vi "Output.vi"(8 "error in (no error)":errorcluster, 10 "SendCMD":bool, 11 "ReadOnlyIIn":T1={"Qref"={"ValveCTR"=refnum, "Error"=refnum}, "UI_EN"=FALSE, "UserEventREF"={"TimeBasedProducer"={"Reg"=refnum, "Ref"=refnum}, "TimeBasedTempRead"={"Reg"=refnum, "Ref"=refnum}}, "UI_REF"=variant, "Paths"={"Log_Dir"=path "", "TempLog"=path "", "WateringLog"=path "", "Error"=path "", "Settings_Dir"=path "", "CFG.ini"=path "", "Plant_Digital_OP"=path "", "TimeTable"=path "", "Consol_Dir"=path "", "Input"=path "", "Output"=path "", "Timeout"=path "", "TimeoutTable"=path "", "Ch_Stat"=path "", "Temp"=path ""}, "PI_REF"={"IO"=enum."Remote", "Interface"=enum."Serial", "LINX Device Config"={"Interface"=enum."Serial", "COM Port"="COM13", "TCP Configuration"={"IP Address"="", "Port"=0}, "Device Family"=1, "Device ID"=1, "Device Name"="myRIO-1900", "TCP Ref"=refnum, "Channels"={"DI"=[0, 1, 2, 3, 4, 5, 6, 7, 8, 9, 10, 11, 12, 13, 14, 15, 16, 17, 18, 19, 20, 21, 22, 23, 24, 25, 26, 27, 28, 29, 30, 31, 32, 33, 34, 35, 36, 37, 38, 39, 40, 41, 42, 43, 44, 45, 46], "DO"=[0, 1, 2, 3, 4, 5, 6, 7, 8, 9, 10, 11, 12, 13, 14, 15, 16, 17, 18, 19, 20, 21, 22, 23, 24, 25, 26, 27, 28, 29, 30, 31, 32, 33, 34, 35, 36, 37, 38, 39, 40, 41, 42, 43, 44, 45, 46], "AI"=[0, 1, 2, 3, 4, 5, 6, 7, 8, 9, 10, 11], "AO"=[], "PWM"=[3, 5, 6, 9, 10], "QE"=[], "UART"=[0, 1], "I2C 2"=[0], "SPI"=[0], "CAN"=[], "Servo"=[], "AI Ref (V)"=0.0, "AI Resolution (Bits)"=0, "AO Ref (V)"=0.0, "AO Resolution (Bits)"=0}}}, "CFG"={"ProducerEn_PC"=FALSE, "Producer_PC_ms"=0, "ProducerEn_PI"=FALSE, "Producer_PI_ms"=0, "TempLogInterval"=15, "SystemResetTime"=0.0}} {"CFG"."SystemResetTime" format="%<%H:%M:%S>t"}) -> (0 "error out":errorcluster)   [LabVIEW 2014, in "Main.lvlib"]
uses:
  Main.lvlib
  TypeDef/ReadOnly.ctl
  ValveCTRL/TypeDef/Queue_Cluster.ctl
  ValveCTRL/TypeDef/States_Enum.ctl
  ValveCTRL/TypeDef/CHs_List.ctl
  TypeDef/EventData.ctl
  <vilib>/MakerHub/LINX/Private/Type Defs/LINX Ref.ctl
  <vilib>/MakerHub/LINX/Private/Type Defs/Platform.ctl
  <vilib>/MakerHub/LINX/Private/Type Defs/Interface.ctl
  <vilib>/MakerHub/LINX/Private/Device/Type Defs/LINX Device Config.ctl
  <vilib>/MakerHub/LINX/Private/Device/Type Defs/TCP Config.ctl
  <vilib>/MakerHub/LINX/Private/Device/Type Defs/Channels.ctl
  Init/ReadInitCFG/TypeDef/CFG_Cluster.ctl
  ValveCTRL/ValveCTRL.lvlib
  <vilib>/MakerHub/LINX/LMH-LINX.lvlib
  <vilib>/MakerHub/LINX/Private/Device/Device.lvlib
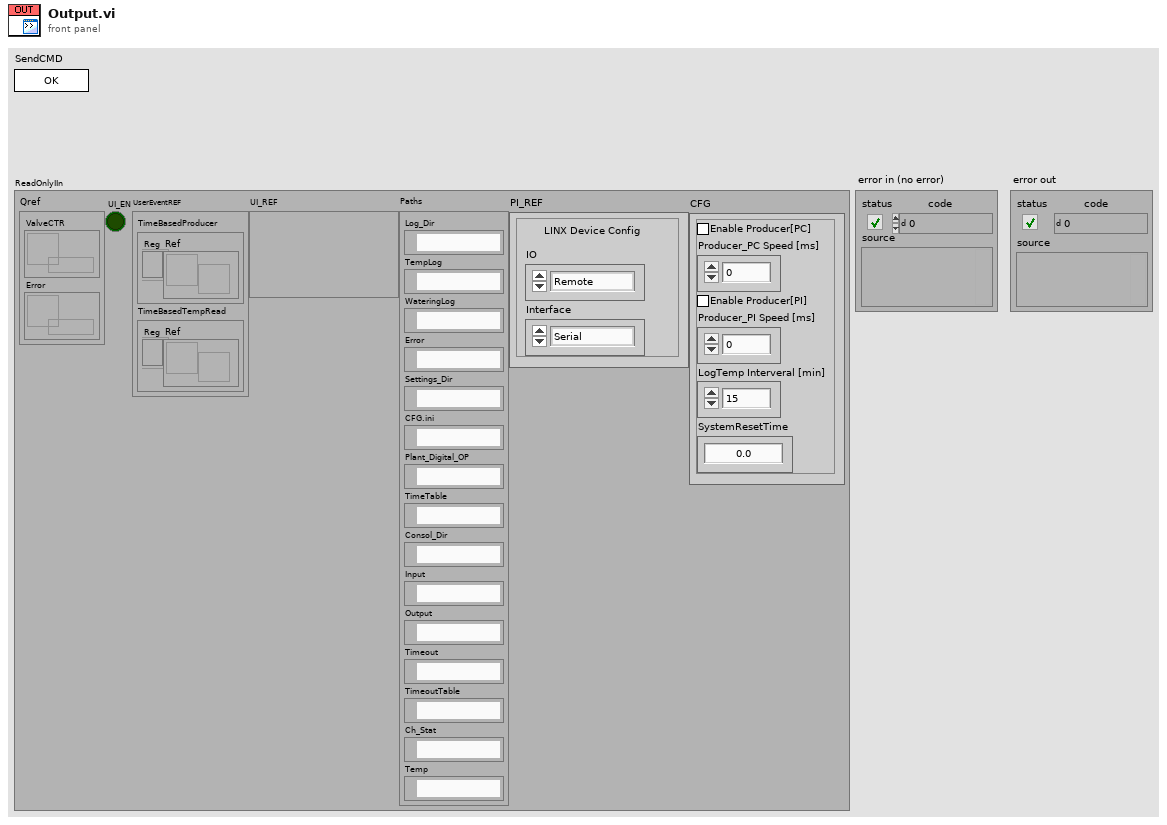
[diagram p1: front panel]
types:
  T1 = typedef "Main.lvlib/ReadOnly.ctl" = cluster{"Qref":cluster{"ValveCTR":refnum<queue>, "Error":refnum<queue>}, "UI_EN":bool, "UserEventREF":cluster{"TimeBasedProducer":cluster{"Reg":refnum<event-registration>, "Ref":refnum<user-event>}, "TimeBasedTempRead":cluster{"Reg":refnum<event-registration>, "Ref":refnum<user-event>}}, "UI_REF":variant, "Paths":cluster{"Log_Dir":path, "TempLog":path, "WateringLog":path, "Error":path, "Settings_Dir":path, "CFG.ini":path, "Plant_Digital_OP":path, "TimeTable":path, "Consol_Dir":path, "Input":path, "Output":path, "Timeout":path, "TimeoutTable":path, "Ch_Stat":path, "Temp":path}, "PI_REF":T2, "CFG":T8}
  T2 = typedef "LMH-LINX.lvlib/LINX Ref.ctl" = cluster{"IO":T3, "Interface":T4, "LINX Device Config":T5}
  T3 = typedef "LMH-LINX.lvlib/Platform.ctl" = enum16{"Remote", "Local"}
  T4 = typedef "LMH-LINX.lvlib/Interface.ctl" = enum16{"Serial", "TCP"}
  T5 = typedef "LMH-LINX.lvlib/Device.lvlib/LINX Device Config.ctl" = cluster{"Interface":T4, "COM Port":refnum<visa-resource-name>, "TCP Configuration":T6, "Device Family":u8, "Device ID":u8, "Device Name":string, "TCP Ref":refnum<k5>, "Channels":T7}
  T6 = typedef "LMH-LINX.lvlib/Device.lvlib/TCP Config.ctl" = cluster{"IP Address":string, "Port":u16}
  T7 = typedef "LMH-LINX.lvlib/Channels.ctl" = cluster{"DI":u8[], "DO":u8[], "AI":u8[], "AO":u8[], "PWM":u8[], "QE":u8[], "UART":u8[], "I2C 2":u8[], "SPI":u8[], "CAN":u8[], "Servo":u8[], "AI Ref (V)":dbl, "AI Resolution (Bits)":u8, "AO Ref (V)":dbl, "AO Resolution (Bits)":u8}
  T8 = typedef "Main.lvlib/CFG_Cluster.ctl" = cluster{"ProducerEn_PC":bool, "Producer_PC_ms":u32, "ProducerEn_PI":bool, "Producer_PI_ms":u32, "TempLogInterval":u32, "SystemResetTime":dbl}
  T9 = enum16{"open", "replace", "create", "open or create", "replace or create", "replace or create with confirmation"}
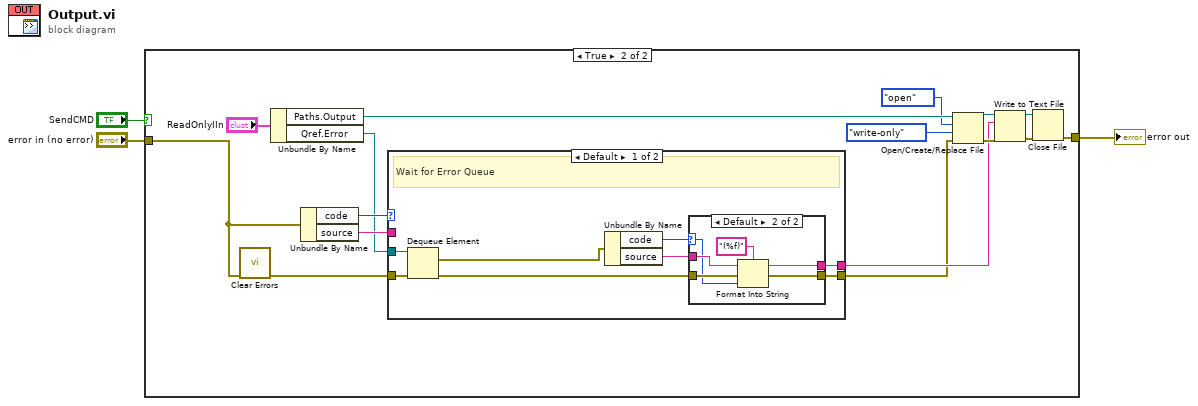
[diagram p0: block diagram]
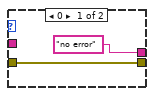
[diagram p3: hidden frame]
diagram:
  n1 = case shown="True" "SendCMD" {
    tunnel: "error in (no error)" -> [w4 w15]
    tunnel: [w4 w11] -> w2
    frame False {
    }
    frame True {
      n2 = call <vilib>:"Clear Errors.vi"("error in (no error)"=w15) -> ("error out"=w6:errorcluster)  [unwired: 5 in, 1 out]
      n3 = Unbundle By Name("ReadOnlyIIn") -> ("Paths.Output"=w19:path, "Qref.Error"=w7:refnum<queue>)
      n4 = Unbundle By Name(w15) -> ("code"=w8:i32, "source"=w9:string)
      n5 = case shown="Default" w8 {
        tunnel: [w25 w38] -> w10
        tunnel: w9 -> [_ w38]
        tunnel: w7 -> [w28 _]
        tunnel: w6 -> [w27 w37]
        tunnel: [w26 w37] -> w5
        frame Default {
          # "Wait for Error Queue"
          n6 = Dequeue Element(queue=w28, error in (no error)=w27) -> (element=w21:errorcluster, error out=w22:errorcluster)  [unwired: 1 in, 2 out]
          n7 = Unbundle By Name(w21) -> ("code"=w24:i32, "source"=w23:string)
          n8 = case shown="Default" w24 {
            selector: w24 -> [_ w31]
            tunnel: ["no error" w34] -> w25
            tunnel: w23 -> [_ w36]
            tunnel: w22 -> [w29 w33]
            tunnel: [w29 w32] -> w26
            frame 0 {
            }
            frame Default {
              n9 = Format Into String(format string="(%f)", initial string=w36, error in=w33, w31) -> (resulting string=w34:string, error out=w32:errorcluster)
            }
          }
        }
        frame 5000 {
          # "Unknown Command"
        }
      }
      n10 = Open/Create/Replace File(file path (use dialog)=w19, error in=w5, operation (0:open)=T9."open", access (0:read/write)=enum16{"read/write", "read-only", "write-only"}."write-only") -> (refnum out=w14:refnum<file>, error out=w16:errorcluster)  [unwired: 2 in, 1 out]
      n11 = Write to Text File(file (use dialog)=w14, text=w10, error in=w16) -> (refnum out=w12:refnum<file>, error out=w13:errorcluster)  [unwired: 1 in, 1 out]
      n12 = Close File(refnum=w12, error in=w13) -> (error out=w11:errorcluster)  [unwired: 1 out]
    }
  }
  "error out" <- w2
